vi "mag-field_get_value.vi"(1 "mag fiel params":T1) -> (0 "field":dbl)   [LabVIEW 2010]
uses:
  mag-field-control.ctl
  type defs - instruments/sweep info.ctl
  type defs - instruments/usage.ctl
  field-info.ctl
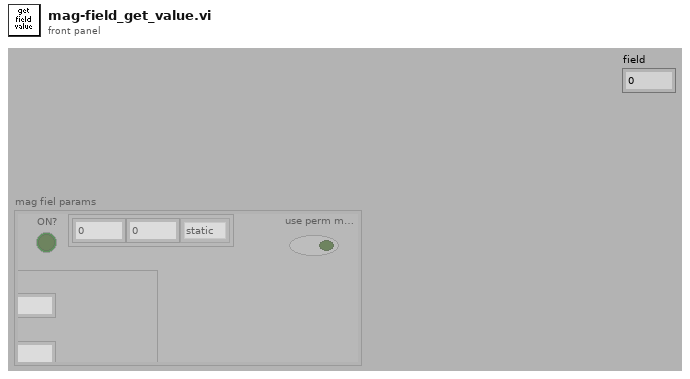
[diagram p1: front panel]
types:
  T1 = typedef "mag-field-control.ctl" = cluster{"mag field":T2, "use perm mode":bool, "field info out":T4, "GPIB adr":string, "driver running?":bool, "ON?":bool, "Coil_Information":cluster{"Max Field 10V Input":dbl, "Waiting time for 0.5mT step":dbl, "Dac_Output_Channel":tag}}
  T2 = typedef "sweep info.ctl" = cluster{"from":sgl, "to":sgl, "type":T3}
  T3 = typedef "usage.ctl" = enum8{"static", "sweep", "step", "step 2", "step 3"}
  T4 = typedef "field-info.ctl" = cluster{"B field (consigne)":dbl, "B field":dbl, "B-field driver (vi reference)":refnum<vi>, "consigne ctrl (driver)":refnum<vi>, "field has arrived (ctrl, driver)":refnum<vi>, "field  (ctrl, driver)":refnum<vi>, "Coil supply":refnum<vi>, "GPIB adress":refnum<vi>}
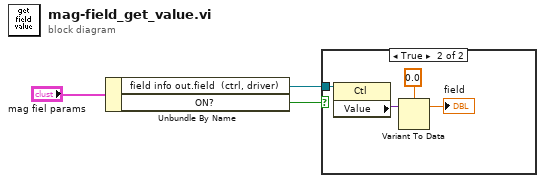
[diagram p0: block diagram]
diagram:
  n1 = Unbundle By Name("mag fiel params") -> ("field info out.field  (ctrl, driver)"=w2:refnum<vi>, "ON?"=w1:bool)
  n2 = case shown="True" w1 {
    tunnel: w2 -> [_ w4]
    frame False {
    }
    frame True {
      n3 = property class="Ctl"(reference=w4) -> ("Value"=w6:variant)  [unwired: 1 in, 2 out]
      n4 = Variant To Data(Variant=w6, type=0.0 ("token")) -> (data=→"field":dbl)  [unwired: 1 in, 1 out]
    }
  }
